vi "Intake Controller.vi"(8 "error in":errorcluster) -> ()   [LabVIEW 2019]
doc: "This VI executes continuously carrying out the current operation and responding to updates or new operations. It will often contain the timing or control code that is difficult to place directly in TeleOp. This VI generally opens all sensors and motors and isolates the rest of the robot code from knowing how the operations are carried out."
uses:
  <vilib>/Rock Robotics/WPI/Framework/Completion Status.ctl
  Intake Setpoints.ctl
  Intake Operations.ctl
  <vilib>/Rock Robotics/WPI/Solenoid/WPI_SolenoidChannel.ctl
  <vilib>/Rock Robotics/WPI/ThirdParty/REV Robotics/SPARK MAX/Typedef/Spark MAX Idle Mode.ctl
  <vilib>/Rock Robotics/WPI/ThirdParty/REV Robotics/SPARK MAX/Typedef/Spark MAX Control Type.ctl
  <vilib>/Rock Robotics/WPI/Solenoid/WPI_SolenoidValue.ctl
  <vilib>/Rock Robotics/WPI/Solenoid/WPI_SolenoidOpenDouble.vi
  <vilib>/Rock Robotics/WPI/Solenoid/WPI_SolenoidSetEnum.vi
  <vilib>/Rock Robotics/Network Tables/NT Write Boolean.vi
panel:
  in  "Interactive Values":T1
  out "Current\nCmd":string
  in  "Buttons":cluster{"Execute Cmd":bool, "Abort Cmd":bool}
  out "Command Timing":cluster{"Start Time (ms)":u32, "Iterations":i32}
  out "Status":T3
  # "Tip: It may be helpful to observe inputs and sensor values.\nYou may also want to display tuning or debugging controls."
  # "Interactive Command: You may fill in the settings for a command\nand schedule it with the Execute button. You can observe and abort\nany command while fine tuning the code for the controller."
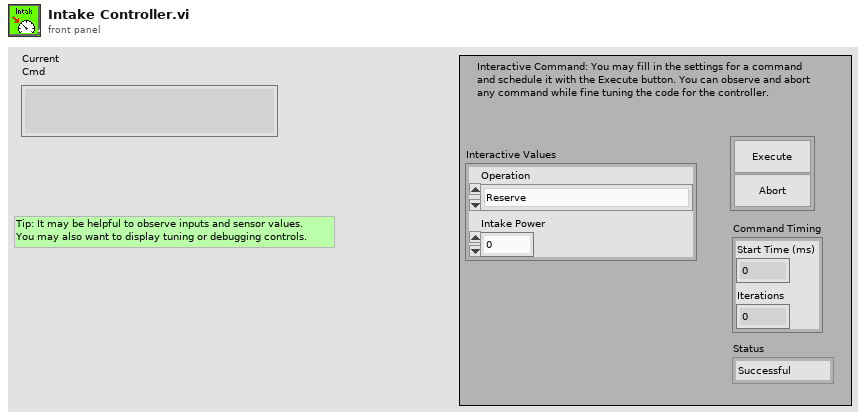
[diagram p1: front panel]
types:
  T1 = typedef "Intake Setpoints.ctl" = cluster{"Operation":T2, "Intake Power":dbl}
  T2 = typedef "Intake Operations.ctl" = enum16{"Reserve", "Read Current", "Immediate", "Extend", "Retract"}
  T3 = typedef "Completion Status.ctl" = enum16{"Successful", "Aborted", "Incomplete"}
  T4 = typedef "WPI_SolenoidChannel.ctl" = enum8{"Solenoid 0", "Solenoid 1", "Solenoid 2", "Solenoid 3", "Solenoid 4", "Solenoid 5", "Solenoid 6", "Solenoid 7", "Invalid"}
  T5 = typedef "WPI_SolenoidDevRef.ctl" = cluster{"DevStatus":errorcluster, "Pneumatics Control Module":u8, "Forward Solenoid Channel":T4, "Reverse Solenoid Channel":T4}
  T6 = typedef "WPI_MotorControlDeviceRef.ctl" = cluster{"DeviceStatus":errorcluster, "Type":T7, "PWM":cluster{"PWM Channel":T8, "DeadBand":T9}, "CAN":cluster{"Device Number":u8, "SetOutput VI Ref":variant, "GetOutput VI Ref":variant, "Enable VI Ref":variant, "Disable VI Ref":variant, "Data":variant}, "Invert":bool, "DIO PWM":cluster{"PWM \"Enable\" Channel":T8, "DIOChannel":T10, "PWM Rate":dbl}}
  T7 = typedef "WPI_MotorControlType.ctl" = enum16{"PWM", "CAN", "DIO PWM"}
  T8 = typedef "FPGA_DIOPWMChannel.ctl" = enum8{"PWM 0", "PWM 1", "PWM 2", "PWM 3", "PWM 4", "PWM 5", "PWM 6", "PWM 7", "PWM 8", "PWM 9", "PWM MXP 0", "PWM MXP 1", "PWM MXP 2", "PWM MXP 3", "PWM MXP 4", "PWM MXP 5", "PWM MXP 6", "PWM MXP 7", "PWM MXP 8", "PWM MXP 9", "Invalid"}
  T9 = typedef "WPI_PWMDeadband.ctl" = cluster{"Name":string, "maxPositivePwm":i32, "minPositivePwm":i32, "centerPwm":i32, "maxNegativePwm":i32, "minNegativePwm":i32, "angularRange":u16}
  T10 = typedef "FPGA_DIOChannel.ctl" = enum8{"DIO 0", "DIO 1", "DIO 2", "DIO 3", "DIO 4", "DIO 5", "DIO 6", "DIO 7", "DIO 8", "DIO 9", "DIO MXP 0", "DIO MXP 1", "DIO MXP 2", "DIO MXP 3", "DIO MXP 4", "DIO MXP 5", "DIO MXP 6", "DIO MXP 7", "DIO MXP 8", "DIO MXP 9", "DIO MXP 10", "DIO MXP 11", "DIO MXP 12", "DIO MXP 13", "DIO MXP 14", "DIO MXP 15", "SPI Port CS1", "SPI Port CS2", "SPI Port CS3", "SPI Port MISO", "SPI Port MOSI", "Invalid"}
  T11 = typedef "Command Status Info.ctl" = cluster{"Name":string, "Status":T3, "notifier out":T12}
  T12 = typedef "Completion Notifier.ctl" = refnum<notifier>
  T13 = cluster{"Current Command":T1, "Command Timing":cluster{"Start Time (ms)":u32, "Iterations":i32}, "Command Arguments":cluster{"Command Info":T11, "Description":string, "Default Command":T1, "queue out":refnum<queue>, "Subsystem Name":string}}
  T14 = typedef "Spark MAX Idle Mode.ctl" = enum16{"Coast", "Brake"}
  T15 = typedef "WPI_SolenoidValue.ctl" = enum16{"Off", "On", "Forward", "Reverse"}
  T16 = typedef "Spark MAX Control Type.ctl" = enum16{"Percent VBus", "Voltage", "Velocity", "Position", "Smart Motion", "Current", "Smart Velocity"}
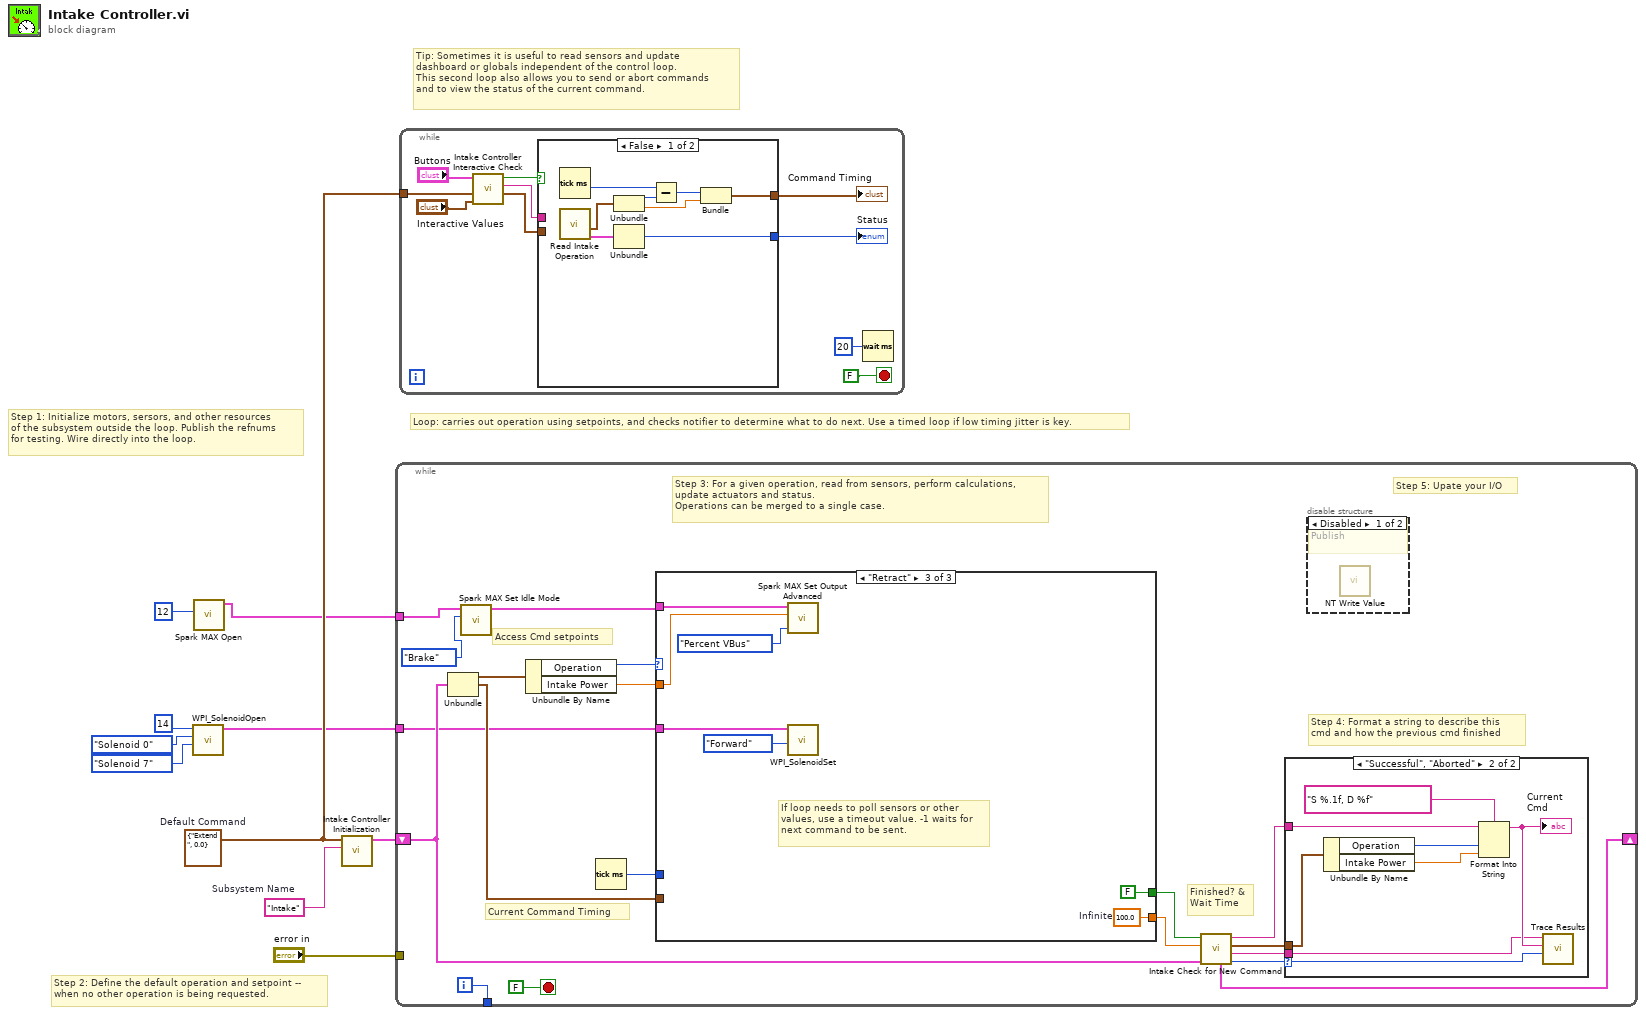
[diagram p0: block diagram]
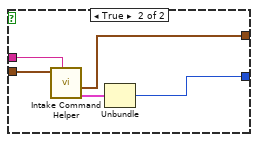
[diagram p2: hidden frame]
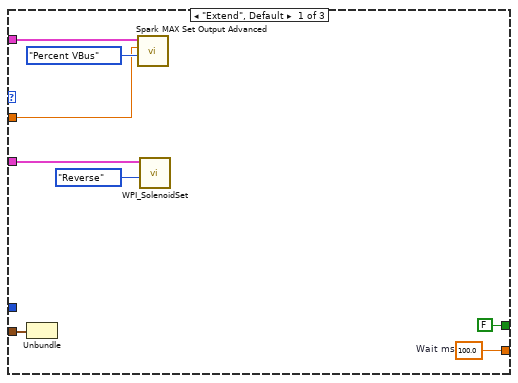
[diagram p5: hidden frame]
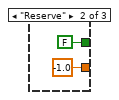
[diagram p6: hidden frame]
diagram:
  w7 = T1 {"Operation"=enum."Extend", "Intake Power"=0.0}  # Default Command
  w8 = "Intake"  # Subsystem Name
  # "Tip: Sometimes it is useful to read sensors and update\ndashboard or globals independent of the control loop.\nThis second loop also allows you to send or abort commands\nand to view the status of the current command."
  # "Step 2: Define the default operation and setpoint --\nwhen no other operation is being requested."
  # "Step 1: Initialize motors, sersors, and other resources\nof the subsystem outside the loop. Publish the refnums\nfor testing. Wire directly into the loop."
  # "Loop: carries out operation using setpoints, and checks notifier to determine what to do next. Use a timed loop if low timing jitter is key."
  n1 = call-poly <vilib>:"WPI_SolenoidOpen.vi"("Reverse Solenoid Channel"=WPI_SolenoidChannel."Solenoid 7", "Forward Solenoid Channel"=WPI_SolenoidChannel."Solenoid 0", "Pneumatics Control Module (0)"=u8 14) -> ("SolenoidDevRef"=w6:T5)  [unwired: 7 in, 1 out]
  n2 = call <vilib>:"Spark MAX Open.vi"("Device Number"=u8 12) -> ("MotorControlDeviceRef"=w1:T6)  [unwired: 9 in, 1 out]
  n3 = call "Intake Controller Initialization.vi"("Subsystem Name"=w8, "Default Command"=w7) -> ("Current Command"=w9:T13)  [unwired: 9 in]
  n4 = while {
    shift-right: [w22] -> _
    shift-left: w9 -> [w15]
    tunnel: [w28] -> _
    tunnel: "error in" -> [_]
    tunnel: w6 -> [w14]
    tunnel: w1 -> [w12]
    i -> [w28]
    stop <- FALSE stop-if-true
    # "Step 5: Upate your I/O"
    # "Step 4: Format a string to describe this\ncmd and how the previous cmd finished"
    # "Current Command Timing"
    # "Access Cmd setpoints"
    # "Finished? &\nWait Time"
    # "Step 3: For a given operation, read from sensors, perform calculations,\nupdate actuators and status.\nOperations can be merged to a single case."
    n5 = Unbundle(w15) -> ("Current Command"=w27:T1, "Command Timing"=w23:cluster{"Start Time (ms)":u32, "Iterations":i32})  [unwired: 1 out]
    n6 = call <vilib>:"Spark MAX Set Idle Mode.vi"("Idle Mode"=Spark_MAX_Idle_Mode."Brake", "MotorControlDeviceRef in"=w12) -> ("MotorControlDeviceRef out"=w11:T6)  [unwired: 8 in, 1 out]
    n7 = Unbundle By Name(w27) -> ("Operation"=w26:T2, "Intake Power"=w25:dbl)
    n8 = Tick Count (ms)() -> (millisecond timer value=w24:u32)
    n9 = case shown="\"Retract\"" w26 {
      tunnel: [w45 -1.0 ("Infinite") w54] -> w20
      tunnel: [FALSE ("ignore previous (F)") FALSE ("ignore previous (F)") FALSE ("ignore previous (F)")] -> w21
      tunnel: w23 -> [w44 _ _]
      tunnel: w25 -> [w38 _ w48]
      tunnel: w24 -> [_ _ _]
      tunnel: w11 -> [w42 _ w50]
      tunnel: w14 -> [w40 _ w51]
      frame "Extend", Default {
        w45 = 100.0  # Wait ms
        n10 = Unbundle(w44) -> ()  [unwired: 2 out]
        n11 = call <vilib>:"Spark MAX Set Output Advanced.vi"("Control Mode"=Spark_MAX_Control_Type."Percent VBus", "Setpoint"=w38, "MotorControlDevRef"=w42) -> ()  [unwired: 7 in, 2 out]
        n12 = call-poly <vilib>:"WPI_SolenoidSet.vi"("Value"=WPI_SolenoidValue."Reverse", "SolenoidDevRef"=w40) -> ()  [unwired: 8 in, 2 out]
      }
      frame "Reserve" {
      }
      frame "Retract" {
        w54 = 100.0  # Infinite
        # "If loop needs to poll sensors or other\nvalues, use a timeout value. -1 waits for\nnext command to be sent."
        n13 = call <vilib>:"Spark MAX Set Output Advanced.vi"("Control Mode"=Spark_MAX_Control_Type."Percent VBus", "Setpoint"=w48, "MotorControlDevRef"=w50) -> ()  [unwired: 7 in, 2 out]
        n14 = call-poly <vilib>:"WPI_SolenoidSet.vi"("Value"=WPI_SolenoidValue."Forward", "SolenoidDevRef"=w51) -> ()  [unwired: 8 in, 2 out]
      }
    }
    n15 = call "Intake Check for New Command.vi"("Current Command"=w15, "Wait time (ms)"=w20, "Finished?"=w21) -> ("Completion"=w16:T3, "Subsystem Name"=w17:string, "Current Command"=w18:T1, "Initial Trace String"=w19:string, "NextCommand"=w22:T13)  [unwired: 4 in]
    n16 = case shown="\"Successful\", \"Aborted\"" w16 {
      selector: w16 -> [_ w37]
      tunnel: w19 -> [_ w33]
      tunnel: w18 -> [_ w34]
      tunnel: w17 -> [_ w30]
      frame "Incomplete", Default {
        # "Continuing current command"
      }
      frame "Successful", "Aborted" {
        # "Report and setup for next command"
        n17 = Unbundle By Name(w34) -> ("Operation"=w36:T2, "Intake Power"=w31:dbl)
        n18 = Format Into String(format string="S %.1f, D %f", initial string=w33, w36, w31) -> (resulting string=w32:string)  [unwired: 1 in, 1 out]
        "Current\nCmd" <- w32
        n19 = call <vilib>:"Trace Results.vi"("Status of previous command"=w37, "Description"=w32, "Subsystem"=w30) -> ()  [unwired: 9 in]
      }
    }
    n20 = disable-structure shown="Disabled" {
      frame Disabled {
        # "Publish"
        n21 = call-poly <vilib>:"NT Write Value.vi"() -> ()  [unwired: 11 in, 1 out]
      }
      frame Enabled {
      }
    }
  }
  n22 = while {
    tunnel: w7 -> [w61]
    stop <- FALSE stop-if-true
    n23 = call "Intake Controller Interactive Check.vi"("Interactive Command in"="Interactive Values", "Default Command"=w61, "Buttons"="Buttons") -> ("Interactive Command out"=w58:T1, "Trace String"=w59:string, "Schedule"=w60:bool)  [unwired: 6 in]
    n24 = case shown="False" w60 {
      tunnel: [w72 w77] -> w57
      tunnel: w58 -> [_ w75]
      tunnel: [w68 w73] -> w56
      tunnel: w59 -> [_ w76]
      frame False {
        n25 = Tick Count (ms)() -> (millisecond timer value=w67:u32)
        n26 = call "Read Intake Operation.vi"() -> ("Command Info"=w65:T11, "SubSystem Data"=w66:T1)  [unwired: 9 in, 1 out]
        n27 = Unbundle(w66) -> ("Operation"=w71:T2, "Intake Power"=w69:dbl)
        n28 = Unbundle(w65) -> ("Status"=w72:T3)  [unwired: 2 out]
        n29 = Subtract(x=w67, y=w71) -> (x-y=w70:u32)
        n30 = Bundle(w70, "Intake Power"=w69) -> (w68:cluster{u32, "Intake Power":dbl})  [unwired: 1 in]
      }
      frame True {
        n31 = call "Intake Command Helper.vi"("Description"=w76, "SubSystem Data"=w75) -> ("Command Info Out"=w74:T11, "Command Timing"=w73:cluster{"Start Time (ms)":u32, "Iterations":i32})  [unwired: 7 in, 1 out]
        n32 = Unbundle(w74) -> ("Status"=w77:T3)  [unwired: 2 out]
      }
    }
    "Status" <- w57
    "Command Timing" <- w56
    n33 = Wait (ms)(milliseconds to wait=u32 20) -> ()  [unwired: 1 out]
  }
